vi "UserEventCaller_1.vi"() -> ()   [LabVIEW 2011]
panel:
  out "Message":string
  out "EventName":T1(ring)
  in  "stop":bool
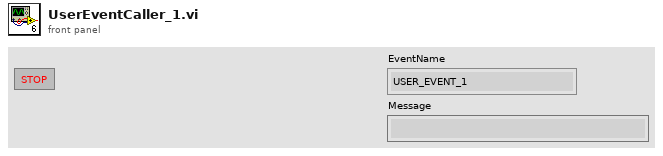
[diagram p1: front panel]
types:
  T1 = enum16{"USER_EVENT_1", "USER_EVENT_2", "USER_EVENT_3", "USER_EVENT_4", "USER_EVENT_5", "USER_EVENT_6", "USER_EVENT_7", "USER_EVENT_8", "USER_EVENT_9", "USER_EVENT_10"}
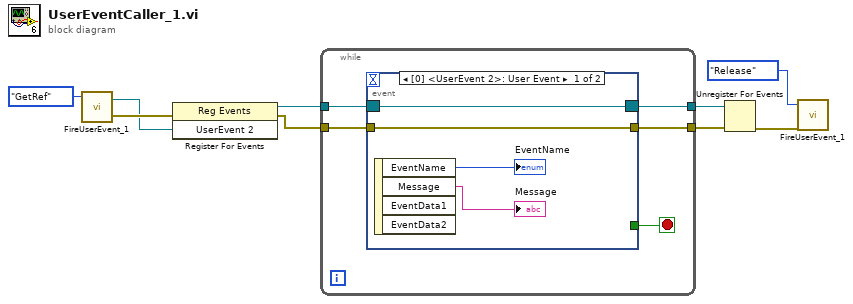
[diagram p0: block diagram]
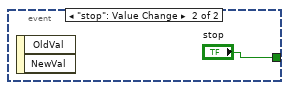
[diagram p2: hidden frame]
diagram:
  n1 = call "FireUserEvent_1.vi"("Enum"=enum16{"GetRef", "Fire", "Release"}."GetRef") -> ("error out"=w8:errorcluster, "UserEvent 2"=w1:refnum<user-event>)  [unwired: 2 in]
  n2 = register-events(error in=w8, w1) -> (reference out=w7:refnum<event-registration>, error out=w5:errorcluster)  [unwired: 1 in]
  n3 = while {
    tunnel: w7 -> [w11]
    tunnel: [w12] -> w6
    tunnel: w5 -> [w14]
    tunnel: [w13] -> w4
    stop <- w10 stop-if-true
    n4 = event shown="[0] <UserEvent 2>: User Event" {
      selector: w11 -> [w17 _]
      dyn-events: [w17 _] -> w12
      timeout: _ -> [_ _]
      tunnel: [w18 _] -> w13
      tunnel: w14 -> [w18 _]
      tunnel: [_ "stop"] -> w10
      event User Event {
        n5 = event-data() -> ("EventName"=→"EventName":T1, "Message"=→"Message":string)  [unwired: 1 in, 2 out]
      }
      event "stop": Value Change {
        n6 = event-data() -> ()  [unwired: 1 in, 2 out]
      }
    }
  }
  n7 = Unregister For Events(event registration refnum=w6, error in=w4) -> (error out=w3:errorcluster)
  n8 = call "FireUserEvent_1.vi"("error in (no error)"=w3, "Enum"=enum16{"GetRef", "Fire", "Release"}."Release") -> ()  [unwired: 1 in, 2 out]
